vi "Lang Create Language File Chinese.vi"(8 "error in (no error)":errorcluster, 11 "LF2R IDE in":refnum<class "Main Panel.lvclass">) -> (0 "error out":errorcluster, 3 "LF2R IDE out":refnum<class "Main Panel.lvclass">)   [LabVIEW 2018, in "Framework.lvlib" / "Framework.lvclass"]
uses:
  Framework/Framework/Framework.lvclass
  Main Panel.lvclass
  0fceaff6-5102-487b-a0d8-62e3909835e7.vi
  <vilib>/JDP Science/JSONtext/Variant to JSON Text.vi
  <vilib>/JDP Science/JSONtext/LVClass Serializer/JSONtext LVClass Serializer.lvclass
  <vilib>/JDP Science/JSONtext/JSONtext.lvlib
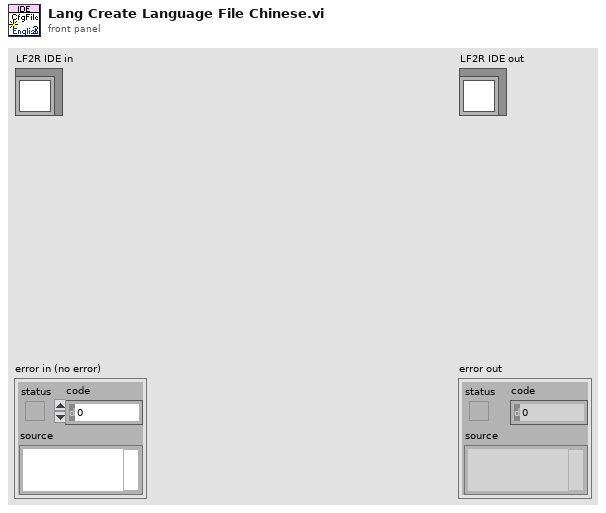
[diagram p1: front panel]
types:
  T1 = enum16{"open", "replace", "create", "open or create", "replace or create", "replace or create with confirmation"}
  T2 = typedef "Framework.lvlib/Framework.lvclass/Const Lang Setting.ctl" = cluster{"Main Panel":T3, "Configuration Window":T16}
  T3 = typedef "Framework.lvlib/Framework.lvclass/Const Lang MainWnd.ctl" = cluster{"Title":T4, "Frame Basic":T6, "Frame Skill":T7, "bp":T8, "w":T9, "b":T10, "i":T11, "o":T12, "c":T13, "Other":T14, "Menu":T15}
  T4 = typedef "Framework.lvlib/Framework.lvclass/Const Lang MainWnd Frame Title.ctl" = cluster{"Frame Num":T5, "Name":T5}
  T5 = typedef "Framework.lvlib/Framework.lvclass/Const Lang Property.ctl" = cluster{"Name":string, "Tip":string, "Description":string}
  T6 = typedef "Framework.lvlib/Framework.lvclass/Const Lang MainWnd Frame Basic.ctl" = cluster{"pic":T5, "state":T5, "wait":T5, "next":T5, "dvx":T5, "dvy":T5, "dvz":T5, "centerx":T5, "centery":T5, "sound":T5}
  T7 = typedef "Framework.lvlib/Framework.lvclass/Const Lang MainWnd Frame Skill.ctl" = cluster{"mp":T5, "hit_a":T5, "hit_d":T5, "hit_j":T5, "hit_Fa":T5, "hit_Ua":T5, "hit_Da":T5, "hit_Fj":T5, "hit_Uj":T5, "hit_Dj":T5, "hit_ja":T5}
  T8 = typedef "Framework.lvlib/Framework.lvclass/Const Lang MainWnd Frame bp.ctl" = cluster{"x":T5, "y":T5}
  T9 = typedef "Framework.lvlib/Framework.lvclass/Const Lang MainWnd Frame w.ctl" = cluster{"kind":T5, "x":T5, "y":T5, "weaponact":T5, "cover":T5, "dvx":T5, "dvy":T5, "dvz":T5, "attacking":T5}
  T10 = typedef "Framework.lvlib/Framework.lvclass/Const Lang MainWnd Frame b.ctl" = cluster{"kind":T5, "x":T5, "y":T5, "w":T5, "h":T5, "index":T5}
  T11 = typedef "Framework.lvlib/Framework.lvclass/Const Lang MainWnd Frame i.ctl" = cluster{"kind":T5, "x":T5, "y":T5, "w":T5, "h":T5, "zwidth":T5, "dvx":T5, "dvy":T5, "dvz":T5, "fall":T5, "arest":T5, "vrest":T5, "bdefend":T5, "injury":T5, "effect":T5, "catchingact 1":T5, "catchingact 2":T5, "caughtact 1":T5, "caughtact 2":T5, "index":T5}
  T12 = typedef "Framework.lvlib/Framework.lvclass/Const Lang MainWnd Frame o.ctl" = cluster{"kind":T5, "x":T5, "y":T5, "action":T5, "dvx":T5, "dvy":T5, "dvz":T5, "oid":T5, "facing":T5}
  T13 = typedef "Framework.lvlib/Framework.lvclass/Const Lang MainWnd Frame c.ctl" = cluster{"kind":T5, "x":T5, "y":T5, "injury":T5, "cover":T5, "vaction":T5, "aaction":T5, "taction":T5, "hurtable":T5, "decrease":T5, "fronthurtact":T5, "backhurtact":T5, "throwvx":T5, "throwvy":T5, "throwvz":T5, "throwinjury":T5, "dircontrol":T5}
  T14 = typedef "Framework.lvlib/Framework.lvclass/Const Lang MainWnd Other.ctl" = cluster{"File Path":T5, "GoTo":T5, "Apply Change":T5, "To Next Frame":T5}
  T15 = typedef "Framework.lvlib/Framework.lvclass/Const Lang MainWnd Menu.ctl" = cluster{"File":T5, "Open File":T5, "Save File":T5, "Exit":T5, "Settings":T5, "Preferences":T5, "Help":T5, "Show Context Help":T5}
  T16 = typedef "Framework.lvlib/Framework.lvclass/Const Lang CfgWnd.ctl" = cluster{"Tab":T17, "Main":T18, "Path":T19, "Image":T20}
  T17 = typedef "Framework.lvlib/Framework.lvclass/Const Lang CfgWnd Tab.ctl" = cluster{"Main Page":T5, "Image Page":T5}
  T18 = typedef "Framework.lvlib/Framework.lvclass/Const Lang CfgWnd Main.ctl" = cluster{"Language":T5, "Save":T5, "Cancel":T5}
  T19 = typedef "Framework.lvlib/Framework.lvclass/Const Lang CfgWnd Path.ctl" = cluster{"Reset":T5, "Path Data":T5, "Path Png":T5}
  T20 = typedef "Framework.lvlib/Framework.lvclass/Const Lang CfgWnd Image.ctl" = cluster{"Center Point":cluster{"Name":T5, "Size":T5, "Color":T5, "Enable":T5}, "bp Point":cluster{"Name":T5, "Size":T5, "Color":T5, "Enable":T5}, "w Point":cluster{"Name":T5, "Size":T5, "Color":T5, "Enable":T5}, "b Box":cluster{"Name":T5, "Fill Color":T5, "Border Color":T5, "Enable":T5}, "i Box":cluster{"Name":T5, "Fill Color":T5, "Border Color":T5, "Enable":T5}, "o Point":cluster{"Name":T5, "Size":T5, "Color":T5, "Enable":T5}, "c Point":cluster{"Name":T5, "Size":T5, "Color":T5, "Enable":T5}}
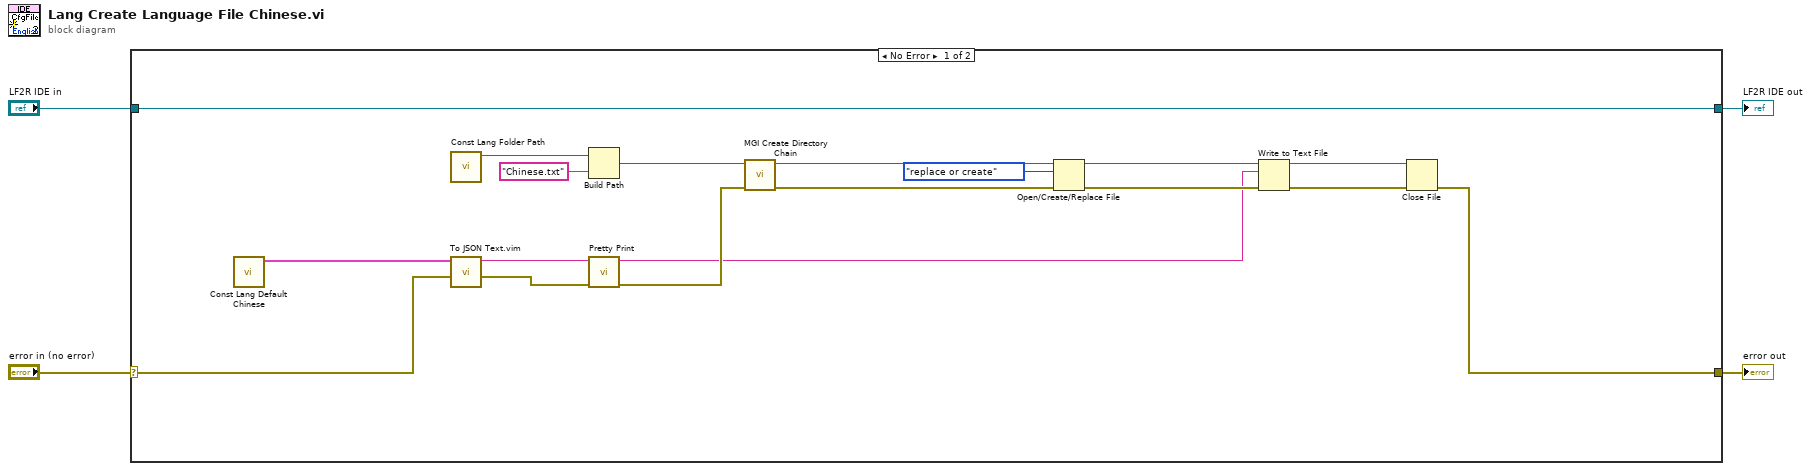
[diagram p0: block diagram]
diagram:
  n1 = case shown="No Error" "error in (no error)" {
    selector: "error in (no error)" -> [w18 w24]
    tunnel: [w9 w24] -> w3
    tunnel: [w22 w23] -> w1
    tunnel: "LF2R IDE in" -> [w22 w23]
    frame No Error {
      n2 = call "Const Lang Default Chinese.vi"() -> ("UI Descriptions"=w5:T2)  [unwired: 11 in]
      n3 = call "Const Lang Folder Path.vi"() -> ("Language Folder Path"=w8:path)  [unwired: 11 in]
      n4 = call "To JSON Text.vim"("error in (no error)"=w18, "Anything"=w5) -> ("error out"=w20:errorcluster, "<JSON>"=w21:string)  [unwired: 8 in]
      n5 = Build Path(base path=w8, name or relative path="Chinese.txt") -> (appended path=w6:path)
      n6 = call <vilib>:"Pretty Print.vi"("error in (no error)"=w20, "JSON"=w21) -> ("error out"=w19:errorcluster, "<JSON>"=w10:string)  [unwired: 7 in, 1 out]
      n7 = call <userlib>:"MGI Create Directory Chain.vi"("Error In"=w19, "Path"=w6) -> ("Error Out"=w11:errorcluster, "Duplicate Path"=w12:path)  [unwired: 8 in]
      n8 = Open/Create/Replace File(file path (use dialog)=w12, error in=w11, operation (0:open)=T1."replace or create") -> (refnum out=w17:refnum<file>, error out=w16:errorcluster)  [unwired: 3 in, 1 out]
      n9 = Write to Text File(file (use dialog)=w17, text=w10, error in=w16) -> (refnum out=w15:refnum<file>, error out=w14:errorcluster)  [unwired: 1 in, 1 out]
      n10 = Close File(refnum=w15, error in=w14) -> (error out=w9:errorcluster)  [unwired: 1 out]
    }
    frame Error {
    }
  }
  "error out" <- w3
  "LF2R IDE out" <- w1
